vi "Test.vi"() -> ()   [LabVIEW 2009]
uses:
  <vilib>/Instr/_visa.llb/VISA Configure Serial Port (Instr).vi
panel:
  in  "Flow Controllers":refnum<visa-resource-name>="COM1"
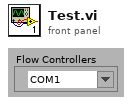
[diagram p1: front panel]
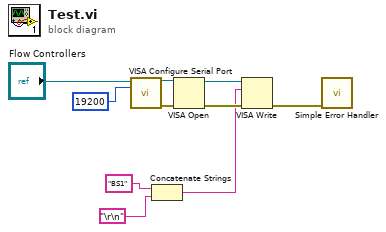
[diagram p0: block diagram]
diagram:
  n1 = call-poly "VISA Configure Serial Port"("VISA resource name"="Flow Controllers", "baud rate (9600)"=19200) -> ("VISA resource name out"=w9:refnum<visa-resource-name>, "error out"=w6:errorcluster)  [unwired: 4 in, 8 out]
  n2 = Concatenate Strings("BS1", "\r\n") -> (w2:string)
  n3 = VISA Open(error in (no error)=w6, VISA resource name=w9) -> (VISA resource name=w7:refnum<visa-resource-name>, error out=w5:errorcluster)  [unwired: 3 in]
  n4 = VISA Write(VISA resource name=w7, write buffer=w2, error in (no error)=w5) -> (error out=w4:errorcluster)  [unwired: 2 out]
  n5 = call <vilib>:"Simple Error Handler.vi"("error in (no error)"=w4) -> ()  [unwired: 4 in, 5 out]
